vi "NXT Camera Test4.vi"() -> ()   [LabVIEW 2016]
uses:
  <vilib>/NXT/Block Support/NXT_InputPort.ctl
  <vilib>/NXT/Block Support/NXT_OutputPort.ctl
  <vilib>/NXT/NXTIO Xnodes/NXTIONodeSubVIs/NXTMoveMotors.vi
  <vilib>/NXT/NXTIO Xnodes/NXTIONodeSubVIs/NXTStopMotors.vi
  <vilib>/NXT/Subs/LVHSConnector.ctl
  <vilib>/NXT/NXTIO Xnodes/AddressXNode/NXTIOAddress.xnode
  <vilib>/NXT/NXTIO Xnodes/NXTIOXNode/NXTIO.xnode
  <vilib>/NXT/LegoClasses/BrickReference/BrickReference.lvclass
panel:
  in  "stop":bool
  out "Power":bool
  out "X Upper Left":u8
  out "X Lower Right":u8
  out "Y Lower Right":u8
  out "Y Upper Left":u8
  out "Count":u8
  out "Color":u8
  in  "Cluster":T1 {"Tracking Mode" items=["Disable Tracking", "Get First Object", "Get n th Object", "Enable Tracking", "Sort Objects  by size", "Sort Objects  by Colors", "Illumination on ", "Illumination Off", "Write Colormap", "Read Colormap", "Line tracking mode", "Object Tracking mode"]}
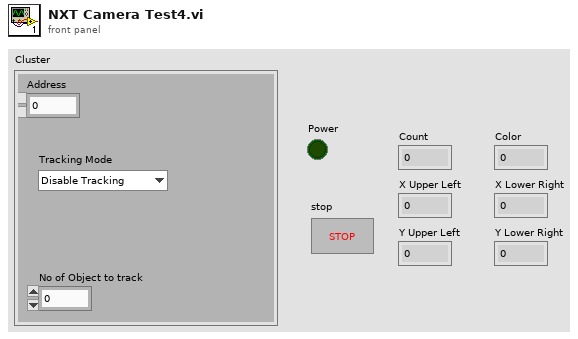
[diagram p1: front panel]
types:
  T1 = cluster{"Address":dbl, "No of Object to track":dbl, "Tracking Mode":u8}
  T2 = cluster{"Tracking Mode":u8, "Object Number to Track":u8, "Address":u8}
  T3 = typedef "NXT_InputPort.ctl" = u32
  T4 = typedef "LVHSConnector.ctl" = refnum<class "BrickReference.lvclass">
  T5 = cluster{"Total Tracked Objects":u8, "Color":u8, "X Upper Left":u8, "Y Upper Left":u8, "X Lower Right":u8, "Y Lower Right":u8, "Status (boolean)":bool}
  T6 = typedef "NXT_OutputPort.ctl" = u8
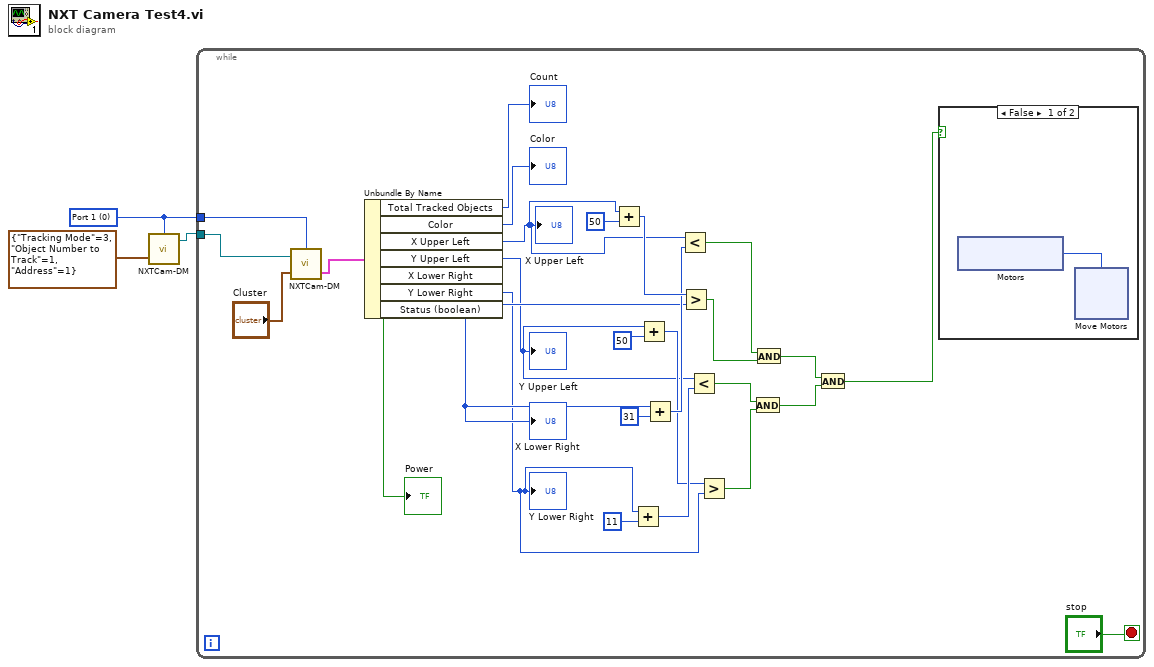
[diagram p0: block diagram]
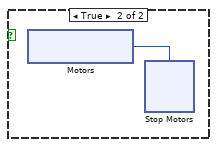
[diagram p2: hidden frame]
diagram:
  w1 = T3 0 items=["Port 1", "Port 2", "Port 3", "Port 4"] ("Input Port")
  n1 = call "NXTCam-DM.vi"("Input of NXTCam"=T2 {"Tracking Mode"=3, "Object Number to Track"=1, "Address"=1}, "Input Port"=w1) -> ("NXT dup"=w3:T4)  [unwired: 1 in, 1 out]
  n2 = while {
    tunnel: w1 -> [w28]
    tunnel: w3 -> [w27]
    stop <- "stop" stop-if-true
    n3 = call "NXTCam-DM.vi"("Input of NXTCam"="Cluster", "NXT"=w27, "Input Port"=w28) -> ("Output of NXTCam"=w6:T5)  [unwired: 1 out]
    n4 = Unbundle By Name(w6) -> ("Total Tracked Objects"=→"Count":u8, "Color"=→"Color":u8, "X Upper Left"=w10:u8, "Y Upper Left"=w9:u8, "X Lower Right"=w11:u8, "Y Lower Right"=w8:u8, "Status (boolean)"=→"Power":bool)
    "X Upper Left" <- w10
    "X Lower Right" <- w11
    "Y Lower Right" <- w8
    "Y Upper Left" <- w9
    n5 = Add(x=w10, y=u8 50) -> (x+y=w17:u8)
    n6 = Add(x=w8, y=u8 11) -> (x+y=w20:u8)
    n7 = Add(x=w9, y=u8 50) -> (x+y=w12:u8)
    n8 = Add(x=w11, y=u8 31) -> (x+y=w14:u8)
    n9 = Less?(x=w10, y=w14) -> (x < y?=w15:bool)
    n10 = Greater?(x=w17, y=w11) -> (0:w18:bool)
    n11 = Less?(x=w9, y=w20) -> (x < y?=w21:bool)
    n12 = Greater?(x=w12, y=w8) -> (0:w23:bool)
    n13 = And(x=w21, y=w23) -> (x .and. y?=w25:bool)
    n14 = And(x=w15, y=w18) -> (x .and. y?=w24:bool)
    n15 = And(x=w24, y=w25) -> (x .and. y?=w4:bool)
    n16 = case shown="False" w4 {
      frame False {
        n17 = xnode "Motors"() -> ("Motor"=w31:T6)
        n18 = xnode "Move Motors"("Motors"=w31) -> ()  [unwired: 2 in, 1 out]
      }
      frame True {
        n19 = xnode "Motors"() -> ("Motor"=w40:T6)
        n20 = xnode "Stop Motors"("Motors"=w40) -> ()  [unwired: 1 in, 1 out]
      }
    }
  }
